vi "DSF.Transceiver.UDP.Constants.vi"   [LabVIEW 2017, in "DSF.Transceiver.UDP.lvlib" / "DSF.Transceiver.UDP.lvclass"]
uses:
  DSF.Transceiver.UDP.lvclass
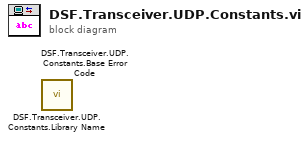
[diagram p0: block diagram]
diagram:
  n1 = call "DSF.Transceiver.UDP.Constants.Library Name.vi"() -> ()  [unwired: 11 in, 1 out]
  n2 = call "DSF.Transceiver.UDP.Constants.Base Error Code.vi"() -> ()  [unwired: 11 in, 1 out]
